vi "UnexpectedDepsCheck1.vi"(6 "StatusIndicator Ref":refnum<vi>, 7 "LibraryNames":string[](array[string]), 8 "error in (no error)":errorcluster, 9 "ActualDependencies File Path":path=path "E:/sw-deps-monitor/Source/ActualDependencies/ActualDepsList.adeps", 10 "BuildSpecs Folder Path":path=path "E:/sw-deps-monitor/Source/BuildSpecs", 11 "Source Folder Path":path=path "E:/sw-deps-monitor/Source") -> (0 "error out":errorcluster)   [LabVIEW 2023, in "Reusables.lvlib"]
uses:
  Reusables/Reusables.lvlib
  Reusables/Typedefs/DepsCheckResult.ctl
  <userlib>/_OpenG.lib/file/file.llb/openg_file.lvlib
  <vilib>/Utility/config.llb/NI_LVConfig.lvlib
panel:
  out "Failures":T1[](array[typedef])
  out "Status Indicator":string
  # "Leave Empty to check all Libraries"
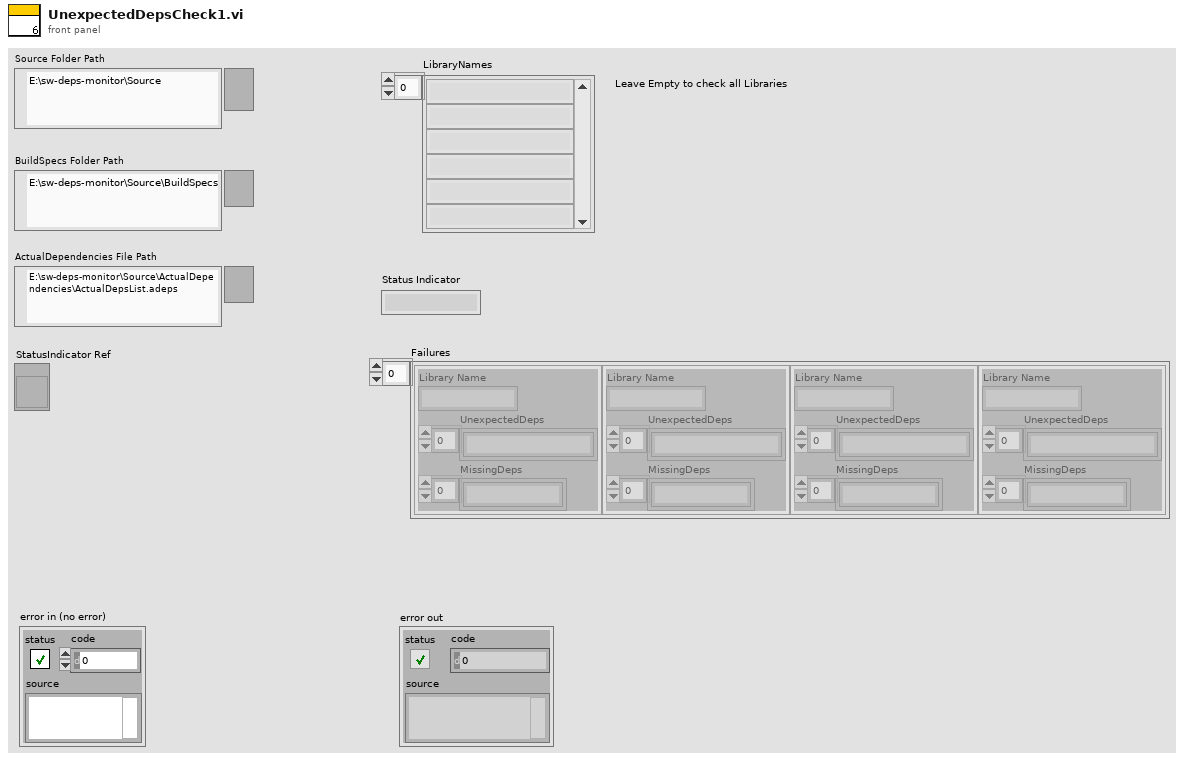
[diagram p1: front panel]
types:
  T1 = typedef "Reusables.lvlib/DepsCheckResult.ctl" = cluster{"Library Name":string, "UnexpectedDeps":string[], "MissingDeps":string[]}
  T2 = typedef "NI_LVConfig.lvlib/Config Data RefNum.ctl" = refnum<k1>
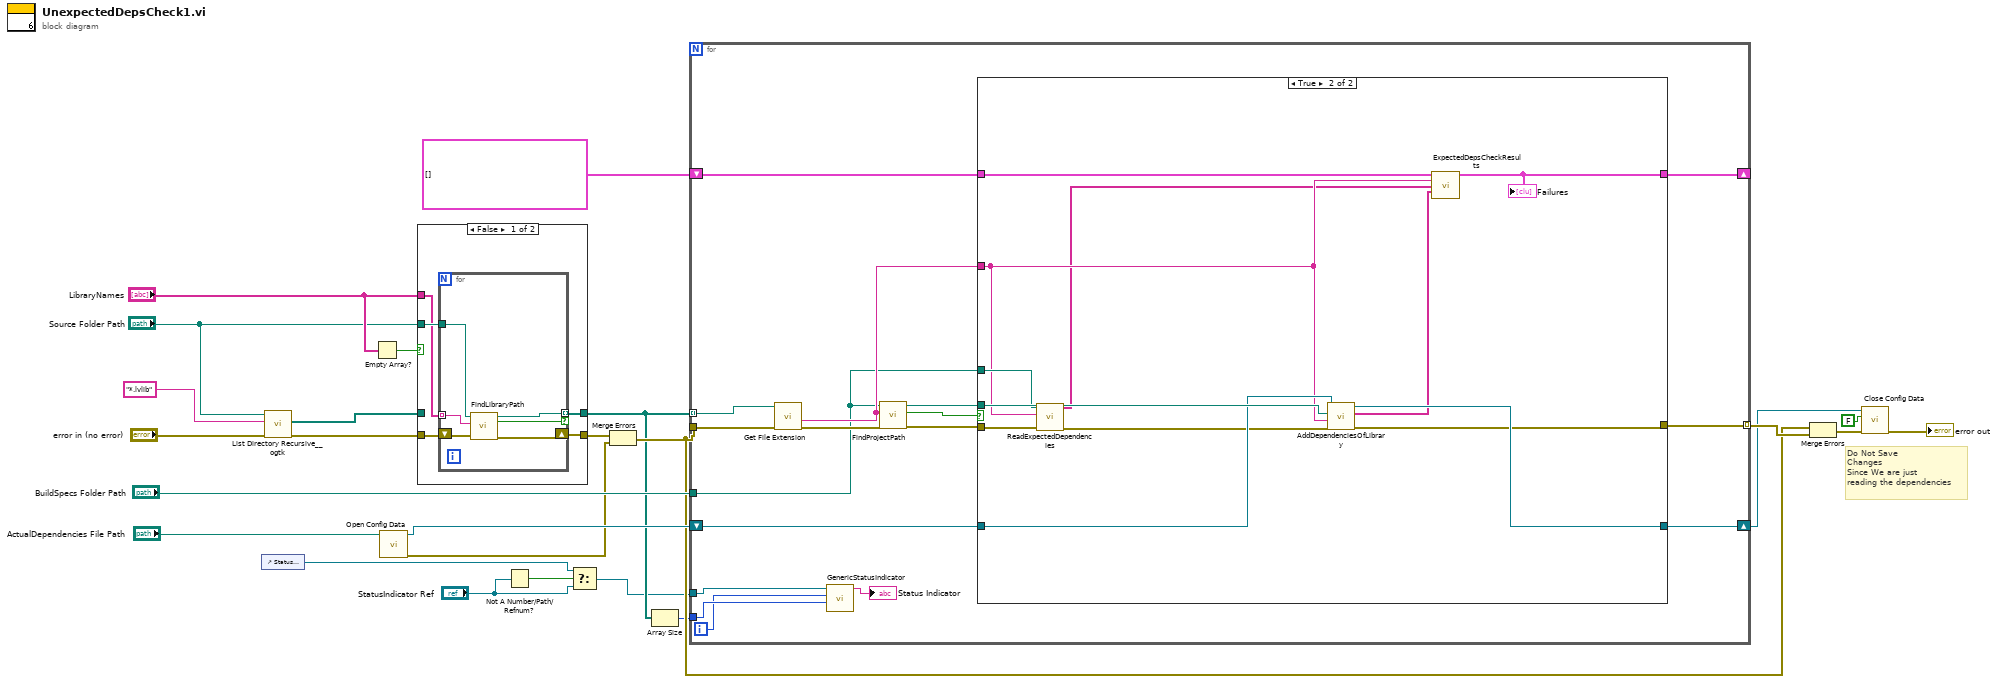
[diagram p0: block diagram]
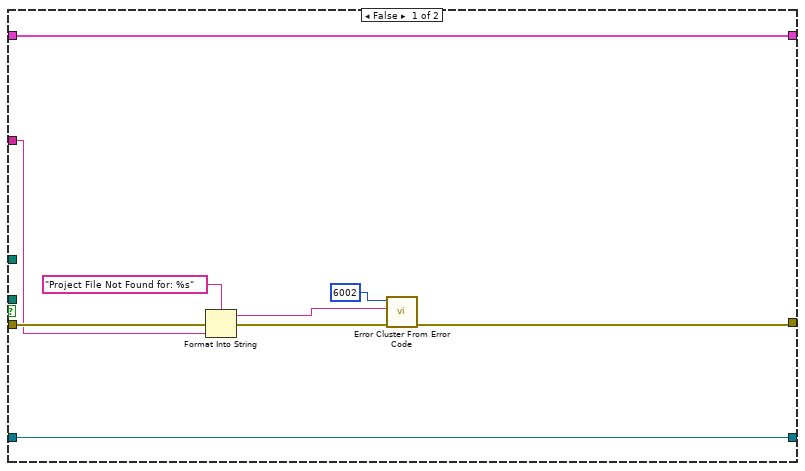
[diagram p3: hidden frame]
diagram:
  # "Do Not Save\nChanges\nSince We are just\nreading the dependencies"
  n1 = control-ref of="Status Indicator"() -> (w5:refnum<vi>)
  n2 = call <userlib>:"List Directory Recursive__ogtk.vi"("error in (no error)"="error in (no error)", "pattern"="*.lvlib", "Path"="Source Folder Path") -> ("error out"=w14:errorcluster, "file paths"=w12:path[])  [unwired: 5 in, 2 out]
  n3 = Empty Array?(array="LibraryNames") -> (empty?=w13:bool)
  n4 = call <vilib>:"Open Config Data.vi"("configuration file path"="ActualDependencies File Path") -> ("error out"=w16:errorcluster, "refnum"=w20:T2)  [unwired: 8 in, 1 out]
  n5 = case shown="False" w13 {
    tunnel: w14 -> [w30 w37]
    tunnel: w12 -> [_ w38]
    tunnel: [w27 w38] -> w8
    tunnel: "LibraryNames" -> [w28 _]
    tunnel: "Source Folder Path" -> [w29 _]
    tunnel: [w26 w37] -> w9
    frame False {
      n6 = for {
        tunnel: w29 -> [w35]
        tunnel: w28 -> [w34] mode=indexing
        shift-right: [w33] -> w26
        shift-left: w30 -> [w36]
        tunnel: [w32] -> w27 mode=indexing if=w31
        n7 = call "FindLibraryPath.vi"("error in (no error)"=w36, "Library Name"=w34, "Source Folder Path"=w35) -> ("error out"=w33:errorcluster, "Found?"=w31:bool, "Library Path"=w32:path)  [unwired: 6 in]
      }
    }
    frame True {
    }
  }
  n8 = Not A Number/Path/Refnum?(number/path/refnum="StatusIndicator Ref") -> (NaN/Path/Refnum?=w6:bool)
  n9 = Select(t=w5, s=w6, f="StatusIndicator Ref") -> (s? t:f=w3:refnum<vi>)
  n10 = Merge Errors(w9, w16) -> (w15:errorcluster)
  n11 = Array Size(array=w8) -> (size(s)=w7:i32)
  n12 = for {
    tunnel: w15 -> [w55]
    tunnel: w8 -> [w53] mode=indexing
    tunnel: "BuildSpecs Folder Path" -> [w41]
    tunnel: [w54] -> w23 mode=indexing
    shift-right: [w47] -> w17
    shift-left: w20 -> [w48]
    tunnel: w3 -> [w45]
    tunnel: w7 -> [w44]
    shift-right: [w39] -> _
    shift-left: T1[] [] -> [w40]
    i -> [w43]
    n13 = call <vilib>:"Get File Extension.vi"("error in (no error)"=w55, "file"=w53) -> ("error out"=w52:errorcluster, "filename without extension"=w46:string)  [unwired: 5 in, 3 out]
    n14 = call "GenericStatusIndicator.vi"("Total"=w44, "Current Iteration"=w43, "String in"=w45) -> ("Status"=→"Status Indicator":string)  [unwired: 8 in]
    n15 = call "FindProjectPath.vi"("error in (no error)"=w52, "Library Name"=w46, "Build Specs Folder Path"=w41) -> ("error out"=w50:errorcluster, "Found?"=w51:bool, "Project Path"=w49:path)  [unwired: 6 in]
    n16 = case shown="True" w51 {
      tunnel: w50 -> [w60 w73]
      tunnel: [w62 w70] -> w54
      tunnel: w49 -> [_ w76]
      tunnel: w48 -> [w64 w75]
      tunnel: [w64 w74] -> w47
      tunnel: w46 -> [w58 w68]
      tunnel: w41 -> [_ w72]
      tunnel: w40 -> [w63 w69]
      tunnel: [w63 w65] -> w39
      frame False {
        n17 = Format Into String(format string="Project File Not Found for: %s", error in=w60, w58) -> (resulting string=w57:string, error out=w56:errorcluster)  [unwired: 1 in]
        n18 = call <vilib>:"Error Cluster From Error Code.vi"("error in (no error)"=w56, "error message (\"\")"=w57, "error code (0)"=6002) -> ("error out"=w62:errorcluster)  [unwired: 6 in]
      }
      frame True {
        n19 = call "ReadExpectedDependencies.vi"("error in (no error)"=w73, "Library Name"=w68, "Build Specs Folder Path"=w72) -> ("error out"=w71:errorcluster, "ExpectedDependencies"=w67:string[])  [unwired: 5 in, 2 out]
        n20 = call "AddDependenciesOfLibrary.vi"("error in (no error)"=w71, "LibraryName"=w68, "Project Path"=w76, "Config Refnum in"=w75) -> ("error out"=w70:errorcluster, "ActualDependencies"=w66:string[], "Config Refnum out"=w74:T2)  [unwired: 5 in]
        n21 = call "ExpectedDepsCheckResults.vi"("ResultsArray"=w69, "Library Name"=w68, "ExpectedDependencies"=w67, "ActualDependencies"=w66) -> ("ResultsArray out"=w65:T1[])  [unwired: 11 in]
        "Failures" <- w65
      }
    }
  }
  n22 = Merge Errors(w15, w23) -> (w19:errorcluster)
  n23 = call <vilib>:"Close Config Data.vi"("error in (no error)"=w19, "write file if changed (T)"=FALSE, "refnum"=w17) -> ("error out"=→"error out":errorcluster)  [unwired: 7 in, 1 out]
